vi "Perceuse.vi"() -> ()   [LabVIEW 2014]
uses:
  Enum.ctl
panel:
  out "# Alarmes detectees":i32
  out "Etat Status":T1
  in  "Nom du fichier":string
  in  "?":bool
  in  "Tension":bool
  in  "Alarme max":u64
  out "Temperature":u64(graph)
  out "Perceuse":T2
  # "Commandes"
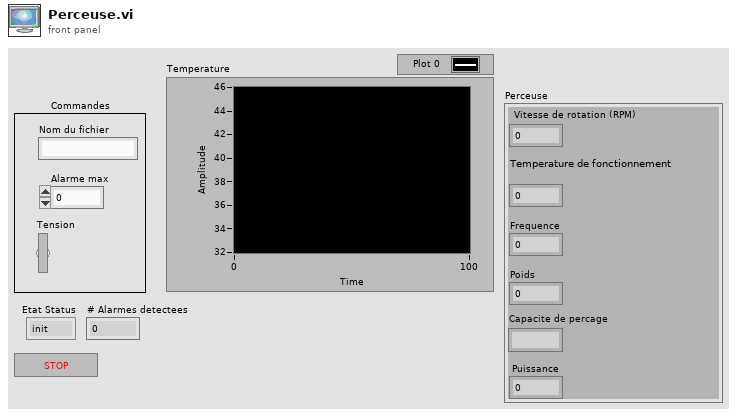
[diagram p1: front panel]
types:
  T1 = typedef "Enum.ctl" = enum16{"init", "run", "close"}
  T2 = cluster{"Vitesse de rotation (RPM)":dbl, "Temperature de fonctionnement":dbl, "Puissance":dbl, "Frequence":dbl, "Poids":dbl, "Capacite de percage":string}
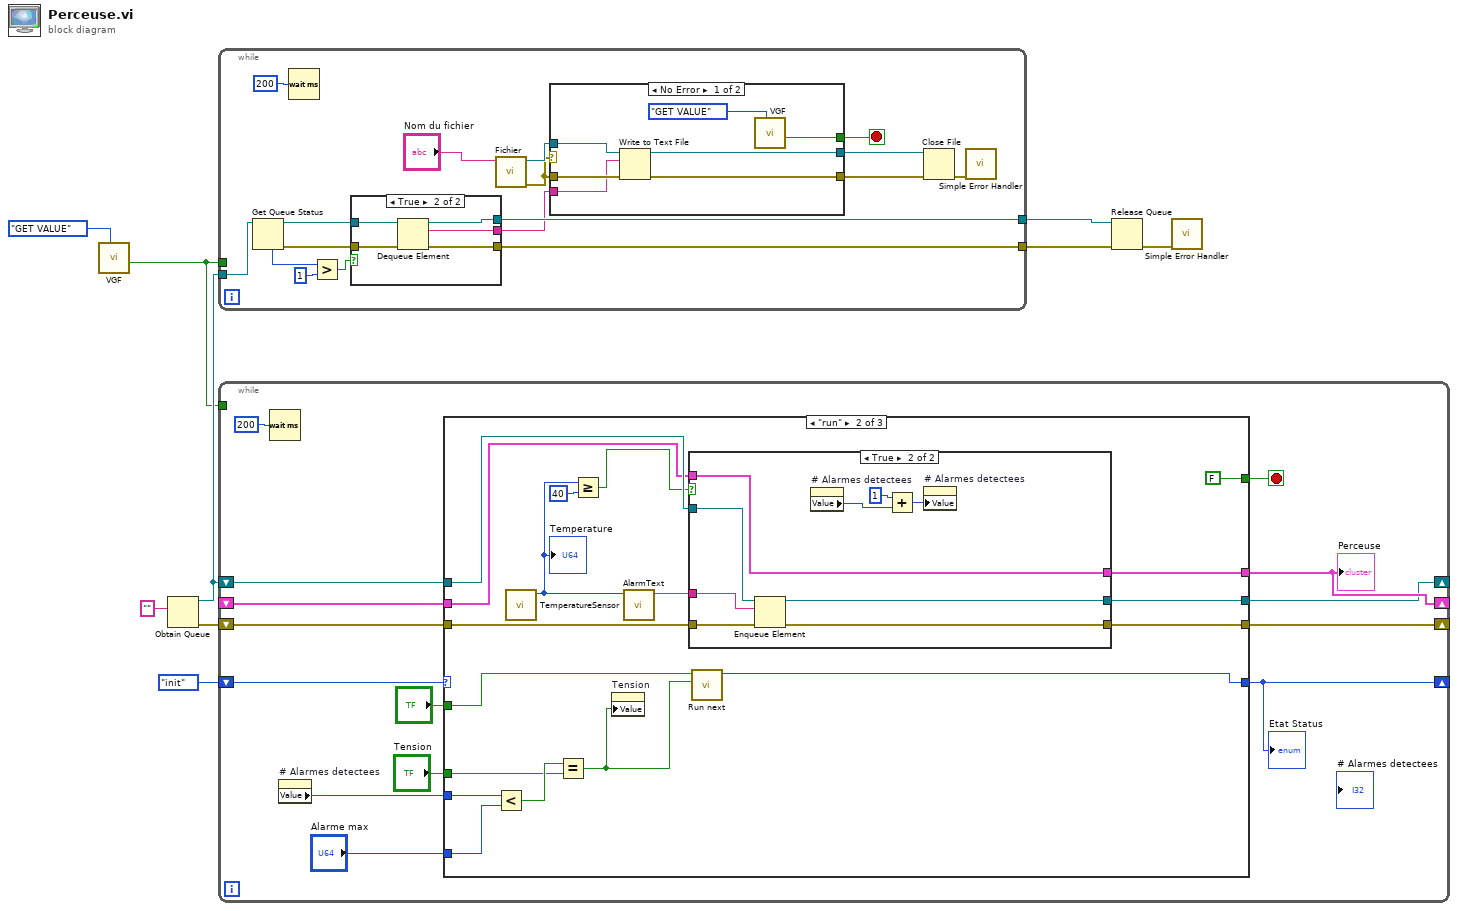
[diagram p0: block diagram]
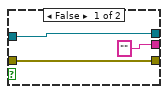
[diagram p2: hidden frame]
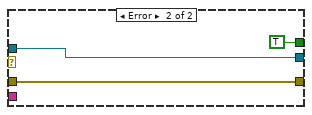
[diagram p3: hidden frame]
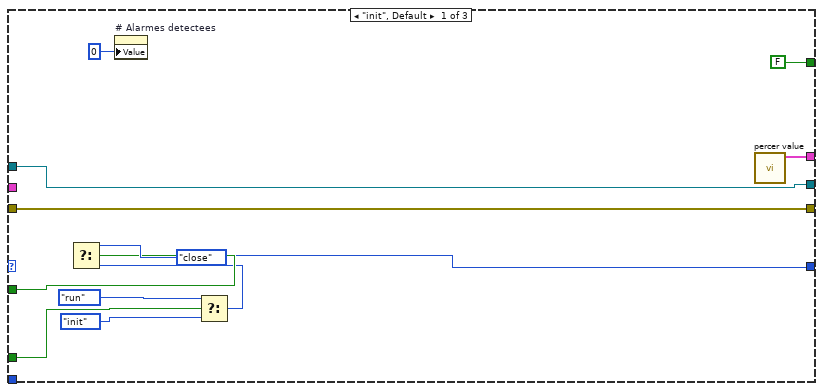
[diagram p4: hidden frame]
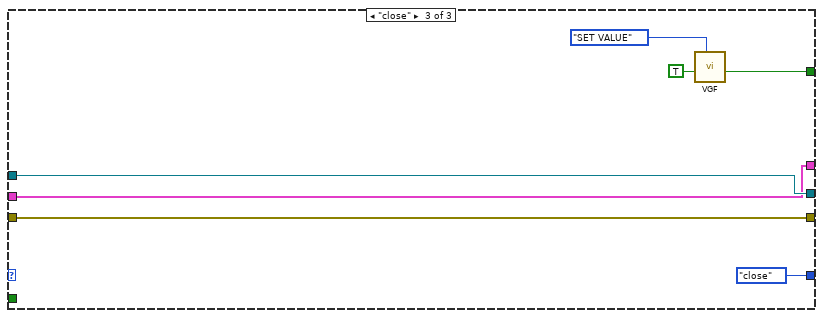
[diagram p6: hidden frame]
diagram:
  n1 = call "VGF.vi"("Enum"=enum16{"GET VALUE", "SET VALUE", "RESET"}."GET VALUE" ("Énum")) -> ("OUT"=w2:bool)  [unwired: 10 in]
  n2 = Obtain Queue(element data type="" ("sin(x)")) -> (queue out=w7:refnum<queue>, error out=w6:errorcluster)  [unwired: 4 in, 1 out]
  n3 = while {
    tunnel: w7 -> [w26]
    tunnel: [w21] -> w5
    tunnel: w2 -> [_]
    tunnel: [w14] -> w1
    stop <- w25 stop-if-true
    n4 = Get Queue Status(queue=w26) -> (queue out=w12:refnum<queue>, error out=w11:errorcluster, # elements in queue=w10:i32)  [unwired: 2 in, 5 out]
    n5 = Wait (ms)(milliseconds to wait=u32 200) -> ()  [unwired: 1 out]
    n6 = Greater?(x=w10, y=1) -> (0:w15:bool)
    n7 = case shown="True" w15 {
      tunnel: [w29 w30] -> w14
      tunnel: [w28 w34] -> w21
      tunnel: w12 -> [w29 w33]
      tunnel: w11 -> [w28 w32]
      tunnel: ["" ("sin(x)") w31] -> w13
      frame False {
      }
      frame True {
        n8 = Dequeue Element(queue=w33, error in (no error)=w32) -> (queue out=w30:refnum<queue>, element=w31:string, error out=w34:errorcluster)  [unwired: 1 in, 1 out]
      }
    }
    n9 = call "Fichier.vi"("Nom de fichier"="Nom du fichier") -> ("error out"=w22:errorcluster, "Byte Stream File out"=w23:refnum<file>)  [unwired: 9 in]
    n10 = case shown="No Error" w22 {
      tunnel: [w36 TRUE ("OUT")] -> w25
      tunnel: w23 -> [w41 w44]
      tunnel: w22 -> [w40 w43]
      tunnel: [w39 w43] -> w17
      tunnel: [w38 w44] -> w18
      tunnel: w13 -> [w35 _]
      frame No Error {
        n11 = Write to Text File(file (use dialog)=w41, text=w35, error in=w40) -> (refnum out=w38:refnum<file>, error out=w39:errorcluster)  [unwired: 1 in, 1 out]
        n12 = call "VGF.vi"("Enum"=enum16{"GET VALUE", "SET VALUE", "RESET"}."GET VALUE" ("Énum")) -> ("OUT"=w36:bool)  [unwired: 10 in]
      }
      frame Error {
      }
    }
    n13 = Close File(refnum=w18, error in=w17) -> (error out=w19:errorcluster)  [unwired: 1 out]
    n14 = call <vilib>:"Simple Error Handler.vi"("error in (no error)"=w19) -> ()  [unwired: 4 in, 5 out]
  }
  n15 = while {
    shift-right: [w45] -> _
    shift-left: Enum."init" -> [w51]
    shift-right: [w57] -> _
    shift-left: _ -> [w58]
    shift-right: [w48] -> _
    shift-left: w7 -> [w50]
    shift-right: [w47] -> _
    shift-left: w6 -> [w49]
    tunnel: w2 -> [_]
    stop <- w52 stop-if-true
    n16 = Wait (ms)(milliseconds to wait=u32 200) -> ()  [unwired: 1 out]
    n17 = property on="# Alarmes detectees" class="DigNum (strict)"() -> ("Value"=w46:i32)  [unwired: 2 in, 2 out]
    n18 = case shown="\"run\"" w51 {
      tunnel: [w61 w73 Enum."close"] -> w45
      tunnel: [w59 w76 w101] -> w57
      tunnel: w58 -> [_ w77 w101]
      tunnel: "Alarme max" -> [_ w87 _]
      tunnel: "Tension" -> [w70 w85 _]
      tunnel: "?" -> [w63 w74 _]
      tunnel: [FALSE FALSE w105] -> w52
      tunnel: [w66 w82 w104] -> w48
      tunnel: w50 -> [w66 w83 w104]
      tunnel: [w65 w80 w103] -> w47
      tunnel: w49 -> [w65 w81 w103]
      tunnel: w46 -> [_ w71 _]
      frame "init", Default {
        n19 = property on="# Alarmes detectees" class="DigNum (strict)"("Value"=0) -> ()  [unwired: 2 in, 2 out]
        n20 = Select(t=Enum."run", s=w70, f=Enum."init") -> (s? t:f=w62:T1)
        n21 = Select(t=Enum."close", s=w63, f=w62) -> (s? t:f=w61:T1)
        n22 = call "percer value.vi"() -> ("Cluster"=w59:cluster{dbl, dbl, dbl, dbl, dbl, string})  [unwired: 11 in]
      }
      frame "run" {
        n23 = Less?(x=w71, y=w87) -> (x < y?=w88:bool)
        n24 = call "TemperatureSensor.vi"() -> ("Output"=w75:u64)  [unwired: 11 in]
        "Temperature" <- w75
        n25 = Equal?(x=w88, y=w85) -> (x = y?=w72:bool)
        n26 = Greater Or Equal?(x=w75, y=u64 40) -> (x >= y?=w79:bool)
        n27 = property on="Tension" class="Bool (strict)"("Value"=w72) -> ()  [unwired: 2 in, 2 out]
        n28 = call "AlarmText.vi"("Input"=w75) -> ("Output"=w78:string)  [unwired: 10 in]
        n29 = case shown="True" w79 {
          tunnel: [w90 w100] -> w82
          tunnel: [w91 w99] -> w80
          tunnel: w81 -> [w91 w97]
          tunnel: w83 -> [w90 w98]
          tunnel: w78 -> [_ w96]
          tunnel: w77 -> [w89 w95]
          tunnel: [w89 w95] -> w76
          frame False {
          }
          frame True {
            n30 = Enqueue Element(queue=w98, element=w96, error in (no error)=w97) -> (queue out=w100:refnum<queue>, error out=w99:errorcluster)  [unwired: 1 in, 1 out]
            n31 = property on="# Alarmes detectees" class="DigNum (strict)"() -> ("Value"=w92:i32)  [unwired: 2 in, 2 out]
            n32 = Add(x=1, y=w92) -> (x+y=w94:i32)
            n33 = property on="# Alarmes detectees" class="DigNum (strict)"("Value"=w94) -> ()  [unwired: 2 in, 2 out]
          }
        }
        n34 = call "Run next.vi"("Boolean 2"=w72, "Boolean"=w74) -> ("Enum"=w73:T1)  [unwired: 9 in]
      }
      frame "close" {
        n35 = call "VGF.vi"("Enum"=enum16{"GET VALUE", "SET VALUE", "RESET"}."SET VALUE" ("Énum"), "STOP"=TRUE) -> ("OUT"=w105:bool)  [unwired: 9 in]
      }
    }
    "Perceuse" <- w57
    "Etat Status" <- w45
  }
  n36 = Release Queue(queue=w1, error in (no error)=w5) -> (error out=w4:errorcluster)  [unwired: 1 in, 2 out]
  n37 = call <vilib>:"Simple Error Handler.vi"("error in (no error)"=w4) -> ()  [unwired: 4 in, 5 out]
